vi "shutdown.vi"() -> ()   [LabVIEW 2023]
panel:
  out "return code":i32
  out "standard error":string
  out "standard output":string
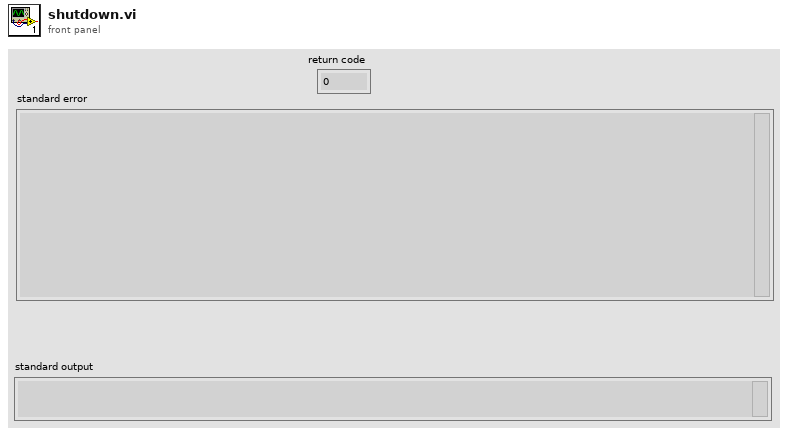
[diagram p1: front panel]
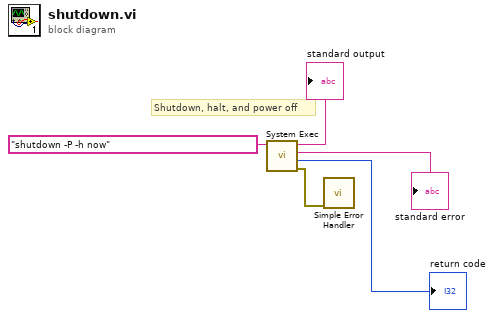
[diagram p0: block diagram]
diagram:
  # "Shutdown, halt, and power off"
  n1 = call <vilib>:"System Exec.vi"("command line"="shutdown -P -h now") -> ("error out"=w1:errorcluster, "return code"=→"return code":i32, "standard error"=→"standard error":string, "standard output"=→"standard output":string)  [unwired: 7 in]
  n2 = call <vilib>:"Simple Error Handler.vi"("error in (no error)"=w1) -> ()  [unwired: 4 in, 5 out]
